vi "Create.vi"(8 "Error In":errorcluster) -> (0 "Error Out":errorcluster, 3 "Display Manager Out":refnum<class "Display Manager.lvclass">)   [LabVIEW 2021, in "Display Manager.lvclass"]
uses:
  Display Manager.lvclass
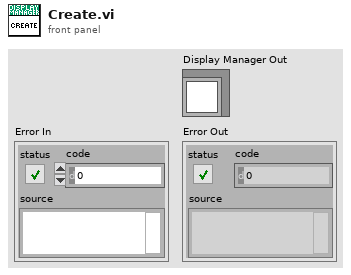
[diagram p1: front panel]
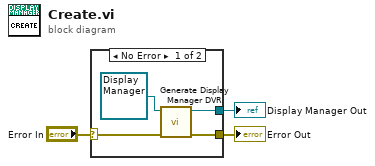
[diagram p0: block diagram]
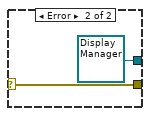
[diagram p2: hidden frame]
diagram:
  n1 = case shown="No Error" "Error In" {
    selector: "Error In" -> [w6 w9]
    tunnel: [w4 refnum<class "Display Manager.lvclass"> refnum ("Screen.lvclass")] -> w3
    tunnel: [w5 w9] -> w1
    frame No Error {
      n2 = call "Generate Display Manager DVR.vi"("Error In"=w6, "Display Manager In"=refnum<class "Display Manager.lvclass"> refnum ("Screen.lvclass")) -> ("Error Out"=w5:errorcluster, "Display Manager Out"=w4:refnum<class "Display Manager.lvclass">)  [unwired: 8 in]
    }
    frame Error {
    }
  }
  "Display Manager Out" <- w3
  "Error Out" <- w1
